vi "Create.vi"(7 "mode settings":variant, 8 "error in":errorcluster, 9 "number of default channels":i32, 10 "channel settings":variant, 11 "ai Arms mode in":refnum<class "Analog Input Arms Mode.lvclass">) -> (0 "error out":errorcluster, 1 "channels":refnum<class "Channel.lvclass">[](array[class]), 3 "ai Arms mode out":refnum<class "Analog Input Arms Mode.lvclass">)   [LabVIEW 2017, in "Scan Engine Scripting.lvlib" / "Analog Input Arms Mode.lvclass"]
uses:
  Analog Input Arms Mode.lvclass
  C:/dev/niveristand-scan-engine-ethercat-custom-device/Custom Device Source/Scripting/Modules/Mode Classes/Analog Input Mode/Analog Input Vrms Mode/Analog Input Mode.lvclass
  Channel Classes/Channel/Channel.lvclass
  Controls/analog channel settings.ctl
  a5d95b34-3fc4-4f73-8903-6a5717812926.vi
  Channel Classes/AI Channel/AI Channel.lvclass
  C:/dev/niveristand-scan-engine-ethercat-custom-device/Custom Device Source/Scripting/Modules/Channel Classes/Channel/Channel.lvclass
  Analog Input Mode/Analog Input Vrms Mode/Analog Input Mode.lvclass
  Scan Engine Scripting.lvlib
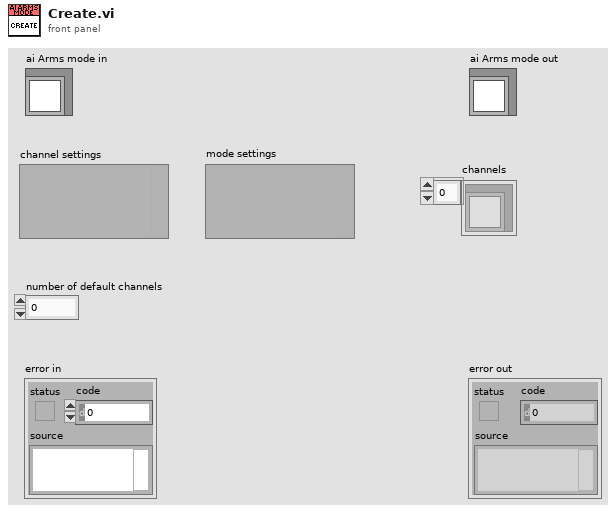
[diagram p1: front panel]
types:
  T1 = typedef "Scan Engine Scripting.lvlib/analog channel settings.ctl" = cluster{"name":string, "default value":dbl}
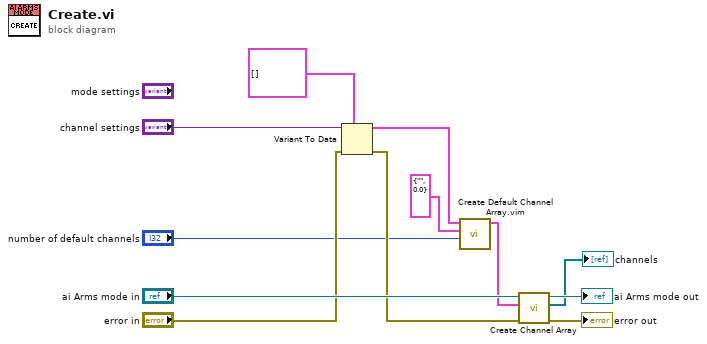
[diagram p0: block diagram]
diagram:
  n1 = Variant To Data(error in="error in", type=T1[] [] ("channel settings"), Variant="channel settings") -> (data=w3:T1[], error out=w6:errorcluster)
  n2 = call "Create Default Channel Array.vim"("number of default channels"="number of default channels", "default settings"=T1 {"name"="", "default value"=0.0} ("channel settings"), "channel settings in"=w3) -> ("channel settings out"=w2:T1[])  [unwired: 8 in]
  n3 = call "Create Channel Array.vi"("error in"=w6, "channel settings"=w2, "analog input mode in"="ai Arms mode in") -> ("error out"=→"error out":errorcluster, "channels"=→"channels":refnum<class "AI Channel.lvclass">[], "analog input mode out"=→"ai Arms mode out":refnum<class "Analog Input Arms Mode.lvclass">)  [unwired: 6 in]
